vi "Save Packets.vi"(4 "SAVE FORMAT":refnum<vi>, 6 "PATH":refnum<vi>, 7 "Headers":string[](array[string]), 8 "error in":errorcluster, 9 "SAVE TO CSV":refnum<vi>, 10 "Packets":refnum<vi>, 11 "Interface Name String":string) -> (0 "error out":errorcluster, 3 "Status Message":string)   [LabVIEW 2025, in "Automotive Ethernet Bus Monitor UI.lvlib"]
doc: "Save the current Package Table to a file."
uses:
  Automotive Ethernet Bus Monitor UI.lvlib
  <vilib>/Utility/file.llb/Write Delimited Spreadsheet (string).vi
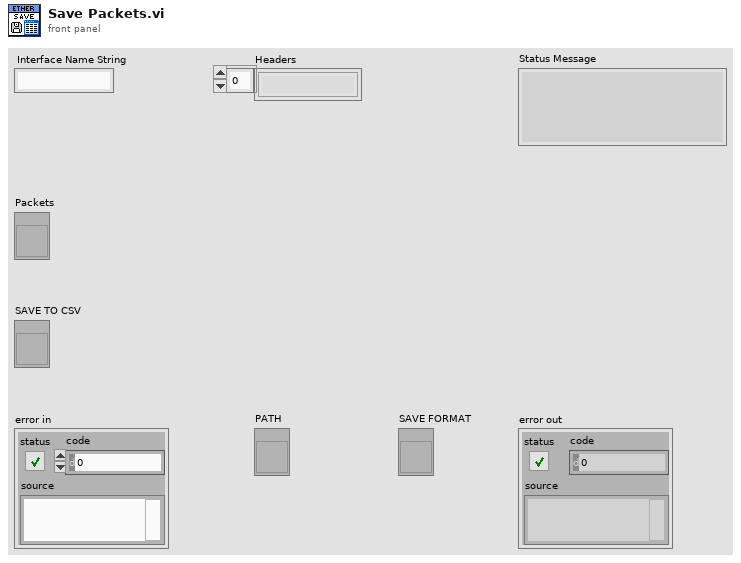
[diagram p1: front panel]
types:
  T1 = enum16{"open", "open or create", "create or replace", "create", "open (read-only)"}
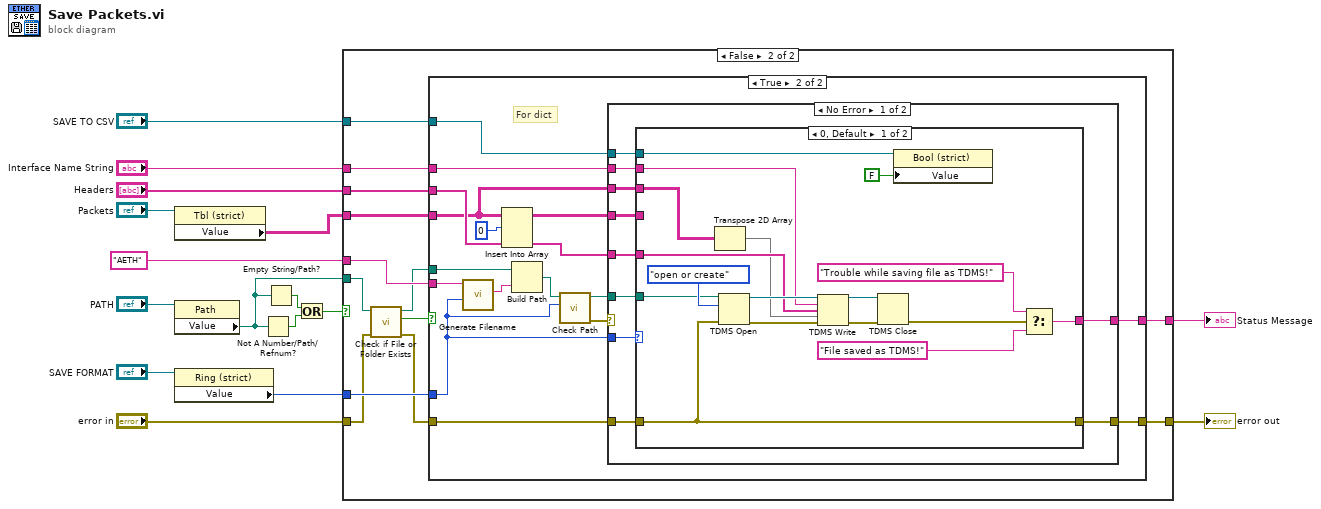
[diagram p0: block diagram]
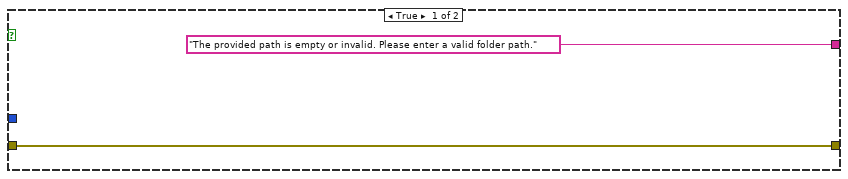
[diagram p2: hidden frame]
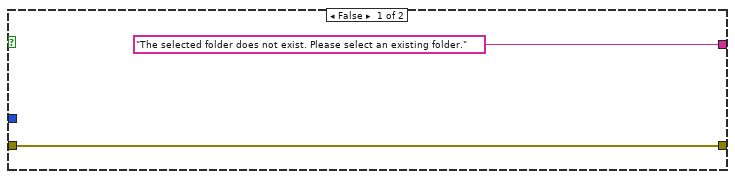
[diagram p3: hidden frame]
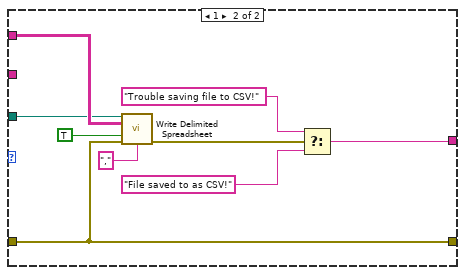
[diagram p4: hidden frame]
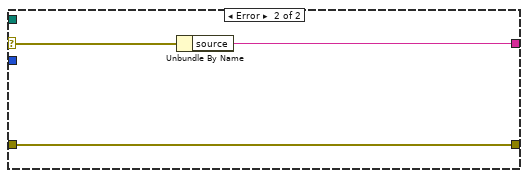
[diagram p5: hidden frame]
diagram:
  n1 = property class="Tbl (strict)"(reference="Packets") -> ("Value"=w5:string[][])  [unwired: 1 in, 2 out]
  n2 = property class="Path"(reference="PATH") -> ("Value"=w15:path)  [unwired: 1 in, 2 out]
  n3 = property class="Ring (strict)"(reference="SAVE FORMAT") -> ("Value"=w16:u16)  [unwired: 1 in, 2 out]
  n4 = Not A Number/Path/Refnum?(number/path/refnum=w15) -> (NaN/Path/Refnum?=w13:bool)
  n5 = Empty String/Path?(string/path=w15) -> (empty?=w12:bool)
  n6 = Or(x=w12, y=w13) -> (x .or. y?=w14:bool)
  n7 = case shown="False" w14 {
    tunnel: [w17 w31] -> w7
    tunnel: "Headers" -> [_ w30]
    tunnel: w5 -> [_ w29]
    tunnel: "error in" -> [w17 w21]
    tunnel: w16 -> [_ w27]
    tunnel: "AETH" ("bustype in") -> [_ w26]
    tunnel: w15 -> [_ w25]
    tunnel: ["The provided path is empty or invalid. Please enter a valid folder path." ("source") w23] -> w11
    tunnel: "Interface Name String" -> [_ w20]
    tunnel: "SAVE TO CSV" -> [_ w19]
    frame True {
    }
    frame False {
      n8 = call <vilib>:"Check if File or Folder Exists.vi"("error in (no error)"=w21, "path"=w25) -> ("error out"=w22:errorcluster, "file or folder exists?"=w28:bool, "dup path"=w24:path)  [unwired: 7 in]
      n9 = case shown="True" w28 {
        tunnel: [w33 w47] -> w31
        tunnel: w30 -> [_ w46]
        tunnel: w29 -> [_ w45]
        tunnel: w22 -> [w33 w40]
        tunnel: w24 -> [_ w39]
        tunnel: w27 -> [_ w38]
        tunnel: w26 -> [_ w37]
        tunnel: ["The selected folder does not exist. Please select an existing folder." ("source") w36] -> w23
        tunnel: w20 -> [_ w35]
        tunnel: w19 -> [_ w34]
        frame False {
        }
        frame True {
          # "For dict"
          n10 = call "Generate Filename.vi"("format  in"=w38, "bustype in"=w37) -> ("filename"=w41:string)  [unwired: 9 in]
          n11 = Insert Into Array(array=w45, index (row)=0, new element=w46) -> (w48:string[][])  [unwired: 1 in]
          n12 = Build Path(base path=w39, name or relative path=w41) -> (appended path=w42:path)
          n13 = call "Check Path.vi"("SAVE TYPE"=w38, "file in"=w42) -> ("Error Out"=w43:errorcluster, "path"=w44:path)  [unwired: 8 in]
          n14 = case shown="No Error" w43 {
            selector: w43 -> [_ w88]
            tunnel: w48 -> [w59 _]
            tunnel: w40 -> [w58 w87]
            tunnel: [w57 w87] -> w47
            tunnel: w46 -> [w56 _]
            tunnel: w45 -> [w55 _]
            tunnel: w44 -> [w54 _]
            tunnel: w38 -> [w53 _]
            tunnel: [w52 w86] -> w36
            tunnel: w35 -> [w51 _]
            tunnel: w34 -> [w50 _]
            frame No Error {
              n15 = case shown="0, Default" w53 {
                tunnel: w59 -> [_ w85]
                tunnel: w58 -> [w64 w78]
                tunnel: w54 -> [w70 w81]
                tunnel: [w64 w78] -> w57
                tunnel: w56 -> [w71 _]
                tunnel: w55 -> [w66 _]
                tunnel: [w63 w77] -> w52
                tunnel: w51 -> [w61 _]
                tunnel: w50 -> [w60 _]
                frame 0, Default {
                  n16 = Transpose 2D Array(2D array=w66) -> (transposed array=w68:string[][])
                  n17 = TDMS Open(8:w64, 10:T1."open or create" ("operation (0:open)"), 11:w70) -> (0:w74:errorcluster, 3:w75:refnum<k34>)  [unwired: 4 in]
                  n18 = TDMS Write(0:w75, 5:w61, 7:w71, 9:w68, 11:w74) -> (4:w72:refnum<k34>, 15:w73:errorcluster)  [unwired: 1 in, 2 out]
                  n19 = TDMS Close(8:w73, 11:w72) -> (0:w62:errorcluster)  [unwired: 1 out]
                  n20 = property class="Bool (strict)"(reference=w60, "Value"=FALSE) -> ()  [unwired: 1 in, 2 out]
                  n21 = Select(t="Trouble while saving file as TDMS!" ("f"), s=w62, f="File saved as TDMS!") -> (s? t:f=w63:string)
                }
                frame 1 {
                  n22 = call-poly <vilib>:"Write Delimited Spreadsheet.vi"("file path (dialog if empty)"=w81, "2D data"=w85, "append to file? (new file:F)"=TRUE, "error in (no error)"=w78, "delimiter (\\t)"="," ("delimiter (\\t)")) -> ("error out"=w80:errorcluster)  [unwired: 9 in, 1 out]
                  n23 = Select(t="Trouble saving file to CSV!" ("f"), s=w80, f="File saved to as CSV!") -> (s? t:f=w77:string)
                }
              }
            }
            frame Error {
              n24 = Unbundle By Name(w88) -> ("source"=w86:string)
            }
          }
        }
      }
    }
  }
  "error out" <- w7
  "Status Message" <- w11
